vi "AccelnetInterface.vi"(8 "Enable":bool, 9 "Clear Faults":bool, 11 "IO Signals":T2) -> (0 "Control word":u16, 3 "Accelnet State":T1)   [LabVIEW 2018]
uses:
  Clusters/IOSignals.ctl
  Clusters/AccelnetState.ctl
panel:
  out "Warning (Bit7)":bool
  out "Switch on disabled (Bit6)":bool
  out "Fault (Bit3)":bool
  out "Operation Enabled (Bit2)":bool
  out "Switched On (Bit1)":bool
  out "Ready to Switch On (Bit0)":bool
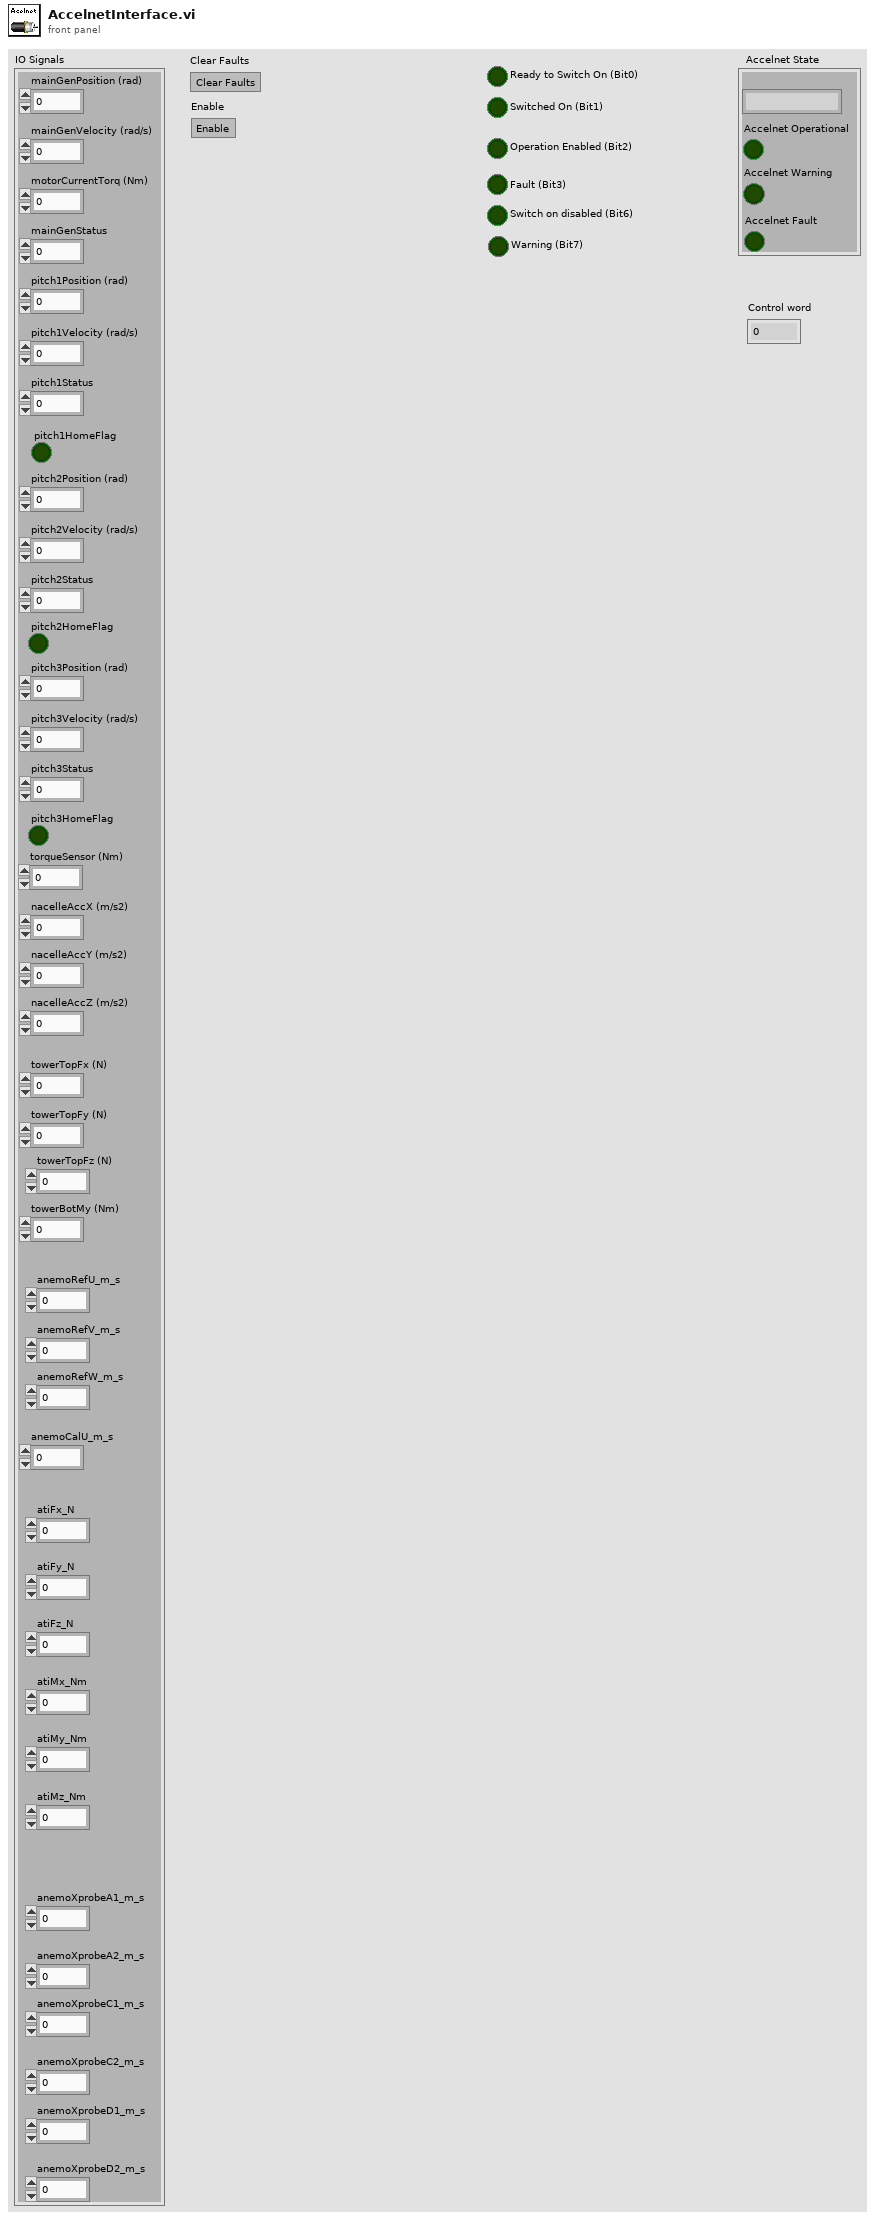
[diagram p1: front panel]
types:
  T1 = typedef "AccelnetState.ctl" = cluster{"State String":string, "Accelnet Warning":bool, "Accelnet Fault":bool, "Accelnet Operational":bool}
  T2 = typedef "IOSignals.ctl" = cluster{"mainGenPosition (rad)":dbl, "motorCurrentTorq (Nm)":dbl, "mainGenVelocity (rad/s)":dbl, "mainGenStatus":u16, "pitch1Position (rad)":dbl, "pitch1Velocity (rad/s)":dbl, "pitch1Status":u16, "pitch2Position (rad)":dbl, "pitch2Velocity (rad/s)":dbl, "pitch2Status":u16, "pitch3Position (rad)":dbl, "pitch3Velocity (rad/s)":dbl, "pitch3Status":u16, "torqueSensor (Nm)":dbl, "nacelleAccX (m/s2)":dbl, "nacelleAccY (m/s2)":dbl, "nacelleAccZ (m/s2)":dbl, "pitch1HomeFlag":bool, "pitch2HomeFlag":bool, "pitch3HomeFlag":bool, "towerTopFx (N)":dbl, "towerTopFy (N)":dbl, "towerTopFz (N)":dbl, "towerBotMy (Nm)":dbl, "anemoRefU_m_s":dbl, "anemoRefV_m_s":dbl, "anemoRefW_m_s":dbl, "atiFx_N":dbl, "atiFy_N":dbl, "atiFz_N":dbl, "atiMx_Nm":dbl, "atiMy_Nm":dbl, "atiMz_Nm":dbl, "anemoCalU_m_s":dbl, "anemoXprobeA1_m_s":dbl, "anemoXprobeA2_m_s":dbl, "anemoXprobeC1_m_s":dbl, "anemoXprobeC2_m_s":dbl, "anemoXprobeD1_m_s":dbl, "anemoXprobeD2_m_s":dbl}
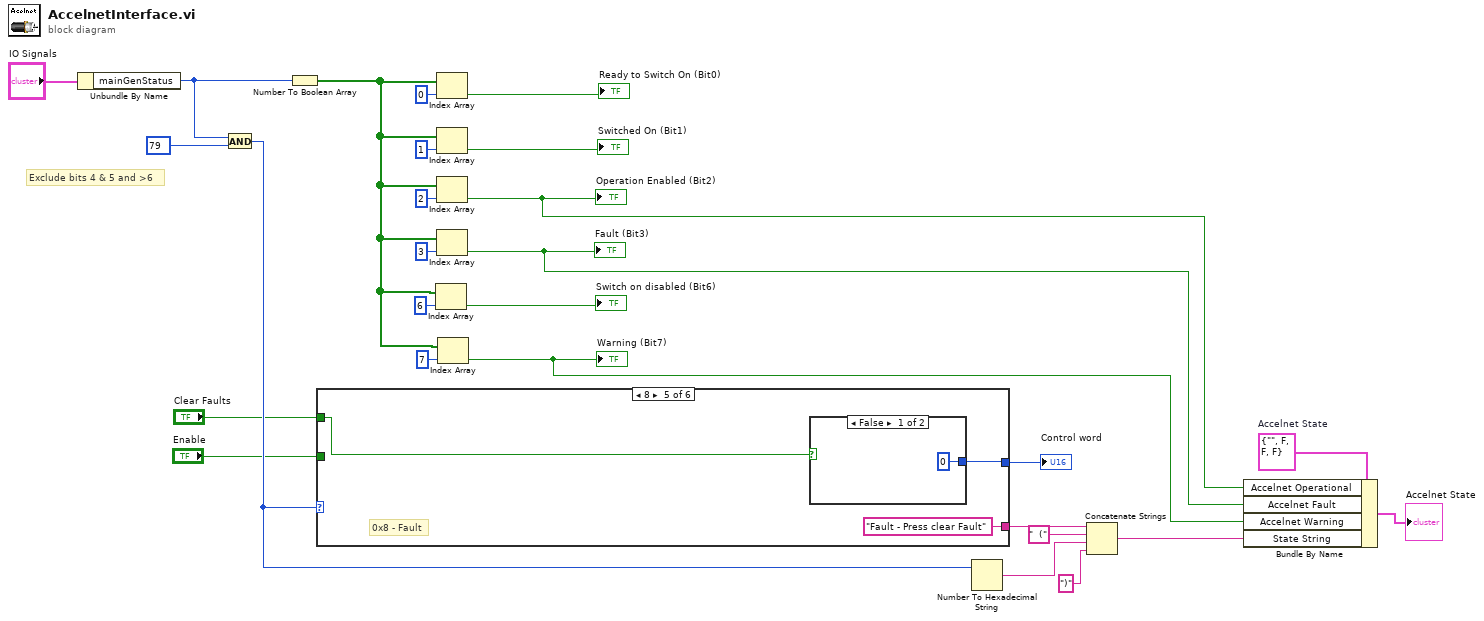
[diagram p0: block diagram]
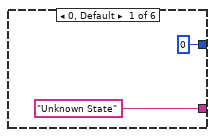
[diagram p2: hidden frame]
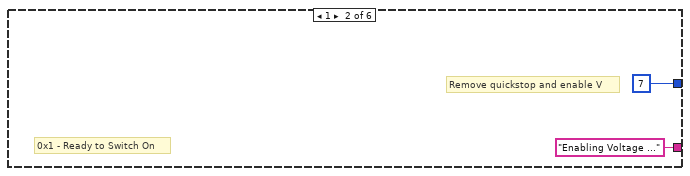
[diagram p3: hidden frame]
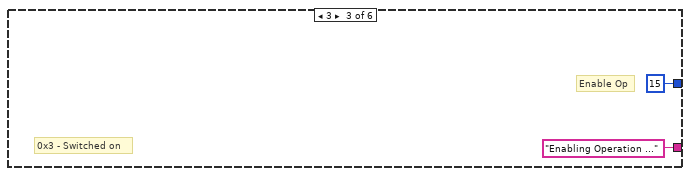
[diagram p4: hidden frame]
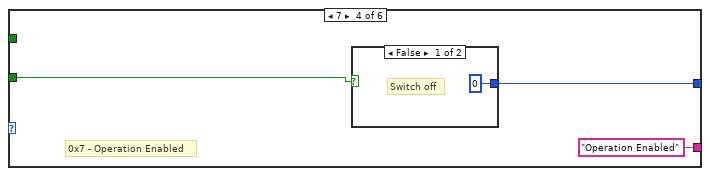
[diagram p5: hidden frame]
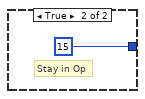
[diagram p6: hidden frame]
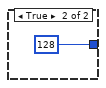
[diagram p7: hidden frame]
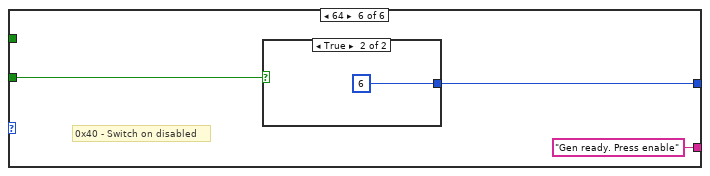
[diagram p8: hidden frame]
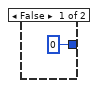
[diagram p9: hidden frame]
diagram:
  w9 = T1 {"State String"="", "Accelnet Warning"=FALSE, "Accelnet Fault"=FALSE, "Accelnet Operational"=FALSE}  # Accelnet State
  # "Exclude bits 4 & 5 and >6"
  n1 = Unbundle By Name("IO Signals") -> ("mainGenStatus"=w12:u16)
  n2 = And(x=w12, y=u16 79) -> (x .and. y?=w10:u16)
  n3 = Number To Boolean Array(number=w12) -> (Boolean array=w18:bool[])
  n4 = case shown="8" w10 {
    tunnel: ["Unknown State" ("AccelNet State") "Enabling Voltage ..." ("AccelNet State") "Enabling Operation ..." ("AccelNet State") "Operation Enabled" ("AccelNet State") "Fault - Press clear Fault" ("AccelNet State") "Gen ready. Press enable" ("AccelNet State")] -> w16
    tunnel: "Enable" -> [_ _ _ w34 _ w45]
    tunnel: [u16 0 ("Control word") u16 7 ("Control word") u16 15 ("Control word") w35 w39 w44] -> w3
    tunnel: "Clear Faults" -> [_ _ _ _ w40 _]
    frame 0, Default {
    }
    frame 1 {
      # "Remove quickstop and enable V"
      # "0x1 - Ready to Switch On"
    }
    frame 3 {
      # "Enable Op"
      # "0x3 - Switched on"
    }
    frame 7 {
      # "0x7 - Operation Enabled"
      n5 = case shown="False" w34 {
        tunnel: [u16 0 ("Control word") u16 15 ("Control word")] -> w35
        frame False {
          # "Switch off"
        }
        frame True {
          # "Stay in Op"
        }
      }
    }
    frame 8 {
      # "0x8 - Fault"
      n6 = case shown="False" w40 {
        tunnel: [u16 0 ("Control word") u16 128 ("Control word")] -> w39
        frame False {
        }
        frame True {
        }
      }
    }
    frame 64 {
      # "0x40 - Switch on disabled"
      n7 = case shown="True" w45 {
        tunnel: [u16 0 ("Control word") u16 6 ("Control word")] -> w44
        frame False {
        }
        frame True {
        }
      }
    }
  }
  "Control word" <- w3
  n8 = Index Array(array=w18, index=6) -> (element=→"Switch on disabled (Bit6)":bool)
  n9 = Index Array(array=w18, index=0) -> (element=→"Ready to Switch On (Bit0)":bool)
  n10 = Index Array(array=w18, index=1) -> (element=→"Switched On (Bit1)":bool)
  n11 = Index Array(array=w18, index=2) -> (element=w1:bool)
  "Operation Enabled (Bit2)" <- w1
  n12 = Index Array(array=w18, index=3) -> (element=w6:bool)
  "Fault (Bit3)" <- w6
  n13 = Index Array(array=w18, index=7) -> (element=w5:bool)
  "Warning (Bit7)" <- w5
  n14 = Number To Hexadecimal String(2:w10) -> (0:w13:string)  [unwired: 1 in]
  n15 = Concatenate Strings(w16, "  (" ("string"), w13, ")" ("string")) -> (w7:string)
  n16 = Bundle By Name(cluster=w9, "Accelnet Operational"=w1, "Accelnet Fault"=w6, "Accelnet Warning"=w5, "State String"=w7) -> (→"Accelnet State":T1)
